vi "sub_ofdm_subcarrier_partitioner.vi"(8 "pilot carrier":i32, 9 "message carrier":i32, 10 "FFT size":i32, 11 "received symbol":cdb[](array[numeric])) -> (0 "pilot subcarriers":cdb[](array[numeric]), 3 "message subcarriers":cdb[](array[numeric]))   [LabVIEW 2014]
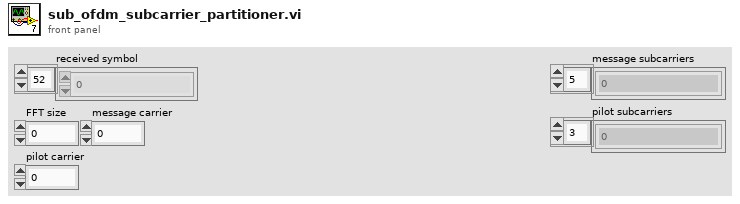
[diagram p1: front panel]
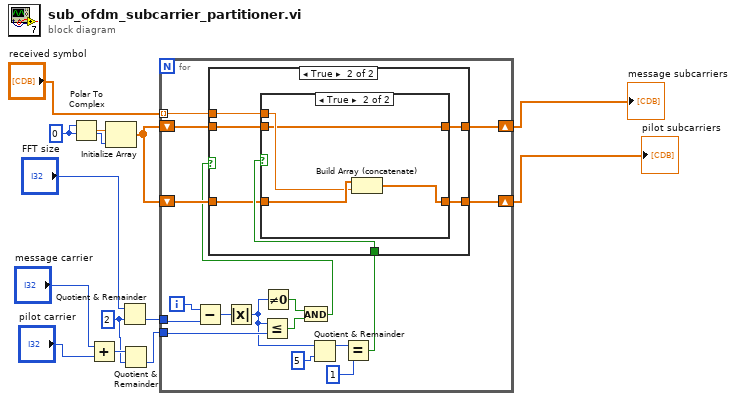
[diagram p0: block diagram]
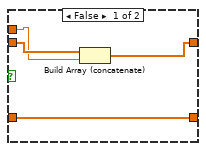
[diagram p3: hidden frame]
diagram:
  w3 = 0
  w2 = 2
  n1 = Polar To Complex(1:w3, 2:w3) -> (0:w7:cdb)
  n2 = Add(x="message carrier", y="pilot carrier") -> (x+y=w9:i32)
  n3 = Initialize Array(w7, w3) -> (w6:cdb[])
  n4 = Quotient & Remainder(x="FFT size", y=w2) -> (floor(x/y)=w13:i32)  [unwired: 1 out]
  n5 = Quotient & Remainder(x=w9, y=w2) -> (floor(x/y)=w1:i32)  [unwired: 1 out]
  n6 = for {
    shift-right: [w29] -> w4
    shift-left: w6 -> [w30]
    shift-right: [w24] -> w5
    shift-left: w6 -> [w28]
    tunnel: w13 -> [w26]
    tunnel: w1 -> [w23]
    tunnel: "received symbol" -> [w17] mode=indexing
    i -> [w27]
    n7 = Subtract(x=w27, y=w26) -> (x-y=w25:i32)
    n8 = Absolute Value(x=w25) -> (abs(x)=w19:i32)
    n9 = Less Or Equal?(x=w19, y=w23) -> (x <= y?=w21:bool)
    n10 = Not Equal To 0?(x=w19) -> (x != 0?=w22:bool)
    n11 = And(x=w22, y=w21) -> (x .and. y?=w20:bool)
    n12 = Quotient & Remainder(x=w19, y=5) -> (x-y*floor(x/y)=w16:i32)  [unwired: 1 out]
    n13 = Equal?(x=w16, y=1) -> (x = y?=w14:bool)
    n14 = case shown="True" w20 {
      tunnel: w30 -> [w31 w36]
      tunnel: [w31 w34] -> w29
      tunnel: w28 -> [w32 w35]
      tunnel: [w32 w33] -> w24
      tunnel: w14 -> [_ w38]
      tunnel: w17 -> [_ w37]
      frame False {
      }
      frame True {
        n15 = case shown="True" w38 {
          tunnel: w37 -> [w40 w45]
          tunnel: w36 -> [w42 w46]
          tunnel: w35 -> [w41 w43]
          tunnel: [w42 w44] -> w34
          tunnel: [w39 w43] -> w33
          frame False {
            n16 = Build Array (concatenate)(w41, w40) -> (w39:cdb[])
          }
          frame True {
            n17 = Build Array (concatenate)(w46, w45) -> (w44:cdb[])
          }
        }
      }
    }
  }
  "message subcarriers" <- w5
  "pilot subcarriers" <- w4
